vi "Dynamic Launcher.vi"(4 "Value":variant, 5 "Wait Until Done":bool, 6 "Control Name":string, 7 "Auto Dispose Reference":bool=TRUE, 8 "error in (no error)":errorcluster, 10 "Dynamic VI's":path, 11 "Folder path":path) -> (0 "error out":errorcluster, 3 "vi reference":refnum<vi>)   [LabVIEW 2017]
doc: "This vi is used to launch the VI's dynamically with Control Input\n\nControl Name- Is Control name exist in the dynamic vi (Leave blank if not required)\nValue - Is for Control exist in the dynamic vi"
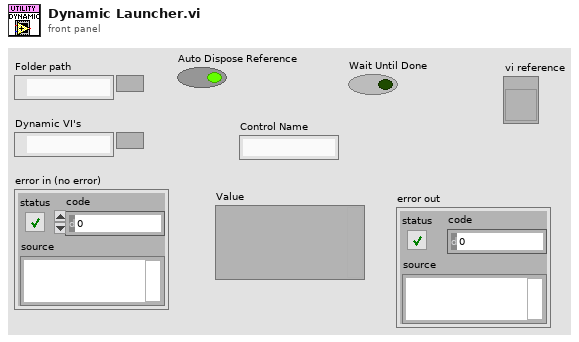
[diagram p1: front panel]
types:
  T1 = enum32{"Bad", "Idle", "Run top level", "Running"}
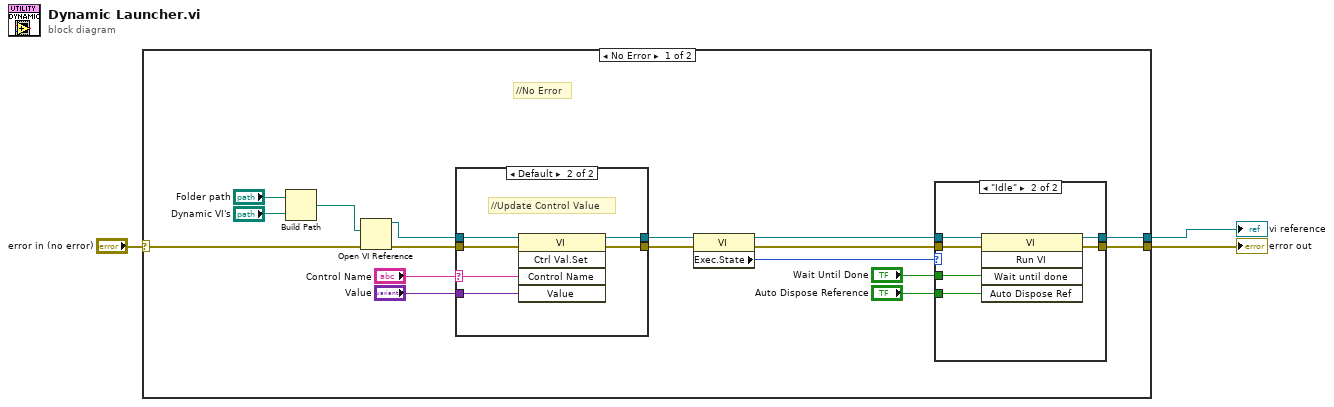
[diagram p0: block diagram]
diagram:
  n1 = case shown="No Error" "error in (no error)" {
    selector: "error in (no error)" -> [w11 w37]
    tunnel: [w20 w37] -> w3
    tunnel: [w4 _] -> w1
    frame No Error {
      # "//No Error"
      n2 = Build Path(base path="Folder path", name or relative path="Dynamic VI's") -> (appended path=w16:path)
      n3 = Open VI Reference(vi path=w16, error in (no error)=w11) -> (vi reference=w9:refnum<vi>, error out=w10:errorcluster)  [unwired: 4 in]
      n4 = case shown="Default" "Control Name" {
        selector: "Control Name" -> [_ w24]
        tunnel: w10 -> [w21 w28]
        tunnel: w9 -> [w22 w27]
        tunnel: [w21 w26] -> w8
        tunnel: [w22 w25] -> w7
        tunnel: "Value" -> [_ w23]
        frame "" {
          # "//Ignore if control name is \nempty"
        }
        frame Default {
          # "//Update Control Value"
          n5 = invoke class="VI" method="Ctrl Val.Set"(reference=w27, error in=w28, "Control Name"=w24, "Value"=w23) -> (reference out=w25:refnum<vi>, error out=w26:errorcluster)  [unwired: 1 in, 3 out]
        }
      }
      n6 = property class="VI"(reference=w7, error in=w8) -> (reference out=w19:refnum<vi>, error out=w18:errorcluster, "Exec.State"=w17:T1)
      n7 = case shown="\"Idle\"" w17 {
        tunnel: w19 -> [w29 w36]
        tunnel: w18 -> [w30 w35]
        tunnel: [w30 w34] -> w20
        tunnel: "Auto Dispose Reference" -> [_ w33]
        tunnel: "Wait Until Done" -> [_ w32]
        tunnel: [w29 w31] -> w4
        frame "Bad", Default {
        }
        frame "Idle" {
          n8 = invoke class="VI" method="Run VI"(reference=w36, error in=w35, "Wait until done"=w32, "Auto Dispose Ref"=w33) -> (reference out=w31:refnum<vi>, error out=w34:errorcluster)  [unwired: 1 in, 3 out]
        }
      }
    }
    frame Error {
      # "//Do Nothing for Error"
    }
  }
  "error out" <- w3
  "vi reference" <- w1
